vi "Authenticate Core.vi"(8 "error in (no error)":errorcluster, 9 "Password":string, 10 "Username":string, 11 "Authentication in":refnum<class "Authentication.lvclass">) -> (0 "error out":errorcluster, 2 "Authenticated?":bool, 3 "Authentication out":refnum<class "Authentication.lvclass">)   [LabVIEW 2016, in "Authentication.lvclass"]
uses:
  Authentication.lvclass
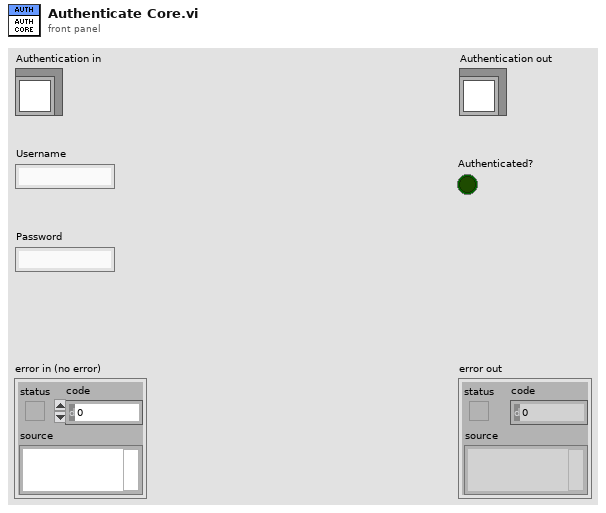
[diagram p1: front panel]
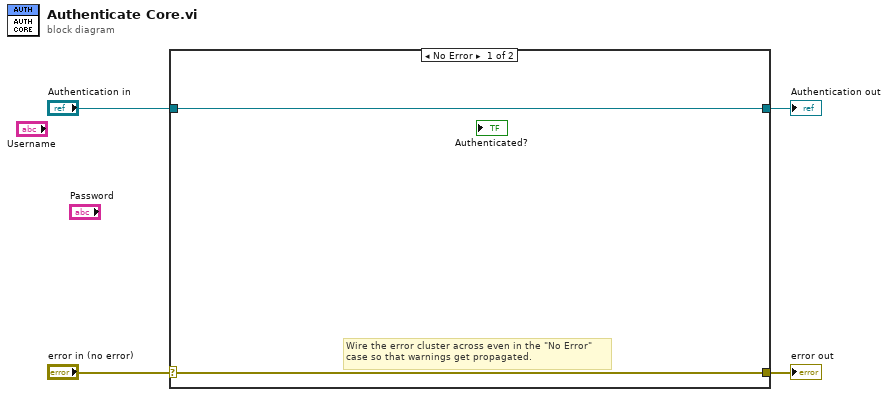
[diagram p0: block diagram]
diagram:
  n1 = case shown="No Error" "error in (no error)" {
    selector: "error in (no error)" -> [w5 w8]
    tunnel: [w5 w8] -> w3
    tunnel: [w6 w7] -> w1
    tunnel: "Authentication in" -> [w6 w7]
    frame No Error {
      # "Wire the error cluster across even in the \"No Error\"\ncase so that warnings get propagated."
    }
    frame Error {
    }
  }
  "error out" <- w3
  "Authentication out" <- w1
